vi "Set Attributes.vi"(7 "Tree ID":string, 8 "Error In":errorcluster, 9 "Attributes Values":variant[](array[variant]), 10 "Attributes Names":string[](array[string]), 11 "Tree Manager":refnum<data-value>) -> (0 "Error Out":errorcluster, 2 "Replaced?":bool[](array[boolean]), 3 "Tree Manager":refnum<data-value>)   [LabVIEW 2017, in "Tree API.lvlib" / "Tree.lvclass"]
doc: "Set variant data array as attributes of the Tree."
uses:
  Tree.lvclass
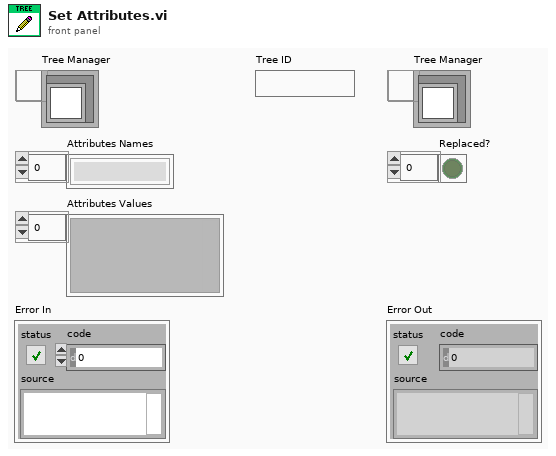
[diagram p1: front panel]
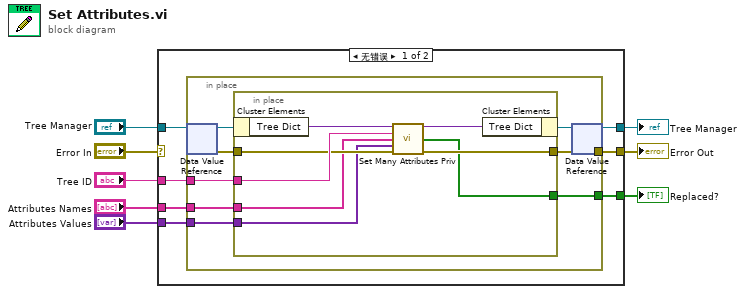
[diagram p0: block diagram]
diagram:
  n1 = case shown="无错误" "Error In" {
    selector: "Error In" -> [_ w32]
    tunnel: "Tree Manager" -> [w15 w33]
    tunnel: [w14 w33] -> w7
    tunnel: [w13 w32] -> w5
    tunnel: "Tree ID" -> [w12 _]
    tunnel: "Attributes Values" -> [w11 _]
    tunnel: "Attributes Names" -> [w10 _]
    tunnel: [w9 _] -> w1
    frame No Error {
      n2 = in-place {
        in-place-border: [w22] -> w13
        in-place-border: w12 -> [w19]
        in-place-border: w11 -> [w18]
        in-place-border: w10 -> [w17]
        in-place-border: [w16] -> w9
        n3 = in-place-dvr #1(w15) -> (w23:refnum<class "Tree.lvclass">, w20:errorcluster)
        n4 = in-place {
          in-place-border: [w27] -> w22
          in-place-border: w20 -> [w28]
          in-place-border: w19 -> [w29]
          in-place-border: w18 -> [w24]
          in-place-border: w17 -> [w25]
          in-place-border: [w26] -> w16
          n5 = in-place-cluster #2(w23) -> ("Tree Dict"=w31:variant)
          n6 = call "Set Many Attributes Priv.vi"("Tree Dictionary Out"=w31, "Unique ID"=w29, "Name"=w25, "Data"=w24, "error in"=w28) -> ("Tree Dictionary Out"=w30:variant, "Replaced?"=w26:bool[], "error out"=w27:errorcluster)  [unwired: 8 in]
          n7 = in-place-cluster #2("Tree Dict"=w30) -> (w21:refnum<class "Tree.lvclass">)
        }
        n8 = in-place-dvr #1(w21) -> (w14:refnum<data-value>)  [unwired: 1 out]
      }
    }
    frame Error {
    }
  }
  "Tree Manager" <- w7
  "Error Out" <- w5
  "Replaced?" <- w1
